vi "refs_parse_format.vi"(7 "string in":string, 8 "error in":errorcluster, 11 "str ind refs":refnum<vi>[](array[refnum])) -> (0 "error out":errorcluster)   [LabVIEW 2013]
uses:
  refs_var.vi
panel:
  out "result string":string
  out "Array":string[](array[string])
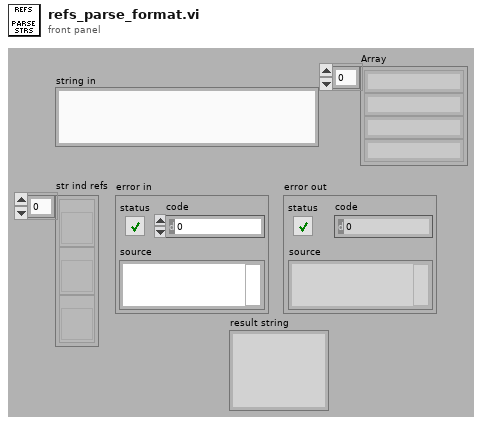
[diagram p1: front panel]
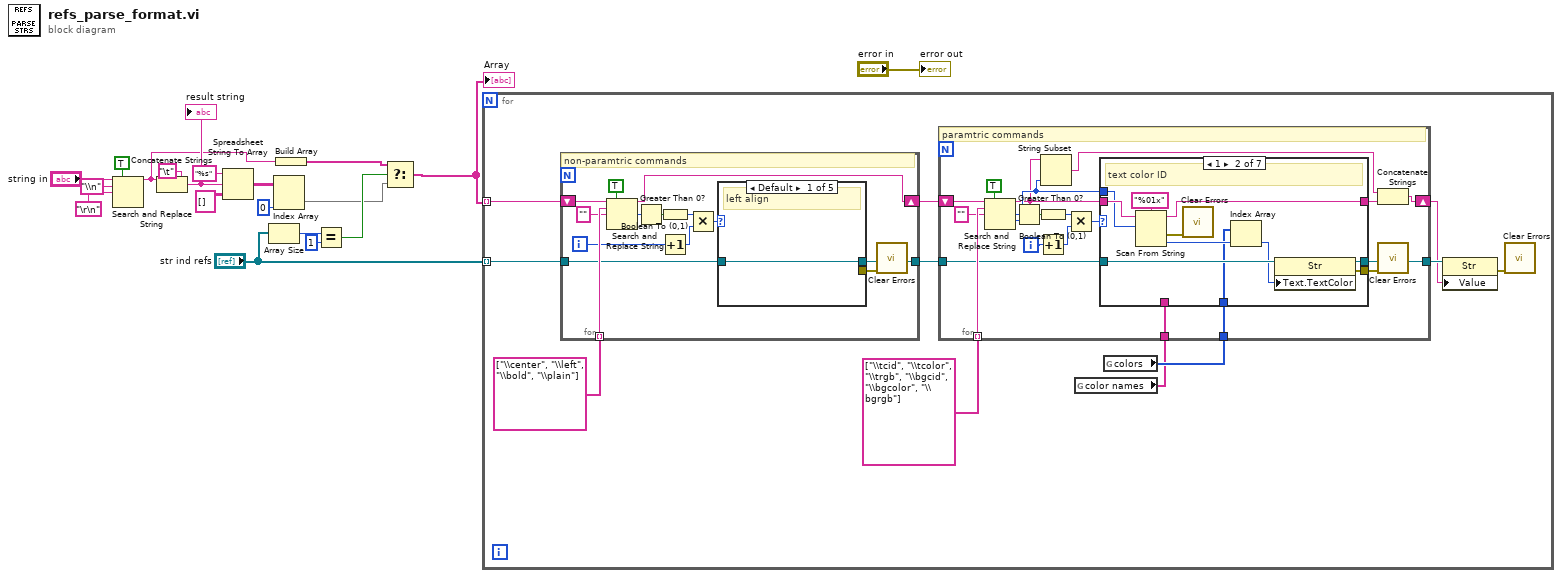
[diagram p0: block diagram]
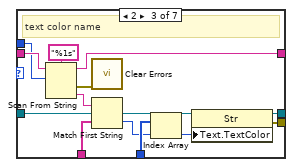
[diagram p3: hidden frame]
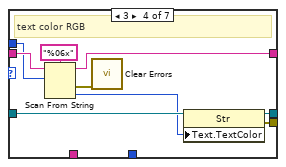
[diagram p4: hidden frame]
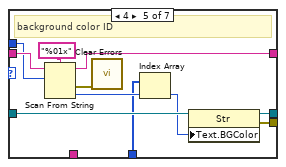
[diagram p5: hidden frame]
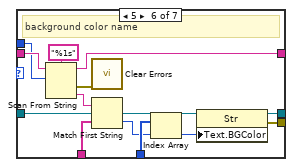
[diagram p6: hidden frame]
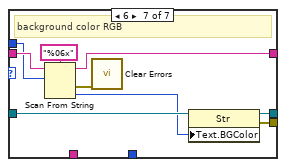
[diagram p7: hidden frame]
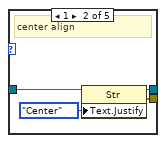
[diagram p8: hidden frame]
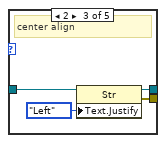
[diagram p9: hidden frame]
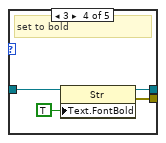
[diagram p10: hidden frame]
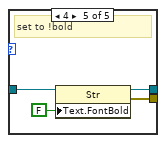
[diagram p11: hidden frame]
diagram:
  n1 = Search and Replace String(replace all?=TRUE ("replace all? (F)"), input string="string in", search string="\\n", replace string="\r\n") -> (result string=w1:string)  [unwired: 4 in, 3 out]
  n2 = Concatenate Strings(w1, "\t") -> (w4:string)
  "result string" <- w4
  n3 = Spreadsheet String To Array(format string="%s", spreadsheet string=w4, array type (2D Dbl)=string[][] []) -> (array=w13:string[][])  [unwired: 1 in]
  n4 = Array Size(array="str ind refs") -> (size(s)=w9:i32)
  n5 = Index Array(array=w13, index (col)=0 ("disabled index (col)")) -> (element=w5:string[])  [unwired: 1 in]
  n6 = Build Array(w1) -> (w3:string[])
  n7 = Equal?(x=w9, y=1) -> (x = y?=w6:bool)
  n8 = Select(t=w3, s=w6, f=w5) -> (s? t:f=w2:string[])
  "Array" <- w2
  n9 = for {
    tunnel: w2 -> [w28] mode=indexing
    tunnel: "str ind refs" -> [w30] mode=indexing
    n10 = for {
      tunnel: string[] ["\\center", "\\left", "\\bold", "\\plain"] -> [w131] mode=indexing
      tunnel: w30 -> [w122]
      tunnel: [w121] -> w27
      shift-right: [w120] -> w26
      shift-left: w28 -> [w132]
      i -> [w125]
      # "non-paramtric commands"
      n11 = Search and Replace String(replace all?=TRUE ("replace all? (F)"), input string=w132, search string=w131, replace string="" ("replace string (\"\")")) -> (result string=w120:string, number of replacements=w128:i32)  [unwired: 4 in, 2 out]
      n12 = Greater Than 0?(x=w128) -> (x > 0?=w127:bool)
      n13 = Boolean To (0,1)(Boolean=w127) -> (0, 1=w126:i16)
      n14 = Increment(x=w125) -> (x+1=w124:i32)
      n15 = Multiply(x=w126, y=w124) -> (x*y=w123:i32)
      n16 = case shown="Default" w123 {
        tunnel: w122 -> [w133 w137 w141 w145 w149]
        tunnel: [w133 w135 w139 w143 w147] -> w121
        tunnel: [_ w134 w138 w142 w146] -> w119
        frame Default {
          # "left align"
        }
        frame 1 {
          # "center align"
          n17 = property class="Str"(reference=w137, "Text.Justify"=enum16{"Left", "Center", "Right"}."Center" ("Text.Justification")) -> (reference out=w135:refnum<vi>, error out=w134:errorcluster)  [unwired: 1 in]
        }
        frame 2 {
          # "center align"
          n18 = property class="Str"(reference=w141, "Text.Justify"=enum16{"Left", "Center", "Right"}."Left" ("Text.Justification")) -> (reference out=w139:refnum<vi>, error out=w138:errorcluster)  [unwired: 1 in]
        }
        frame 3 {
          # "set to bold"
          n19 = property class="Str"(reference=w145, "Text.FontBold"=TRUE ("Text.Font:Bold")) -> (reference out=w143:refnum<vi>, error out=w142:errorcluster)  [unwired: 1 in]
        }
        frame 4 {
          # "set to !bold"
          n20 = property class="Str"(reference=w149, "Text.FontBold"=FALSE ("Text.Font:Bold")) -> (reference out=w147:refnum<vi>, error out=w146:errorcluster)  [unwired: 1 in]
        }
      }
      n21 = call <vilib>:"Clear Errors.vi"("error in (no error)"=w119) -> ()  [unwired: 6 in, 1 out]
    }
    n22 = global read "refs_var.vi" "color names"() -> (w22:string[])
    n23 = global read "refs_var.vi" "colors"() -> (w24:u32[])
    n24 = for {
      tunnel: string[] ["\\tcid", "\\tcolor", "\\trgb", "\\bgcid", "\\bgcolor", "\\bgrgb"] -> [w49] mode=indexing
      tunnel: w27 -> [w40]
      tunnel: [w39] -> w23
      shift-right: [w34] -> w21
      shift-left: w26 -> [w50]
      tunnel: w24 -> [w38]
      tunnel: w22 -> [w32]
      i -> [w43]
      # "paramtric commands"
      n25 = Search and Replace String(replace all?=TRUE ("replace all? (F)"), input string=w50, search string=w49, replace string="" ("replace string (\"\")")) -> (result string=w36:string, number of replacements=w46:i32, offset past replacement=w37:i32)  [unwired: 4 in, 1 out]
      n26 = Greater Than 0?(x=w46) -> (x > 0?=w45:bool)
      n27 = Boolean To (0,1)(Boolean=w45) -> (0, 1=w44:i16)
      n28 = Increment(x=w43) -> (x+1=w42:i32)
      n29 = String Subset(string=w36, length (rest)=w37) -> (substring=w33:string)  [unwired: 1 in]
      n30 = Multiply(x=w44, y=w42) -> (x*y=w41:i32)
      n31 = case shown="1" w41 {
        tunnel: w40 -> [w52 w63 w76 w85 w96 w109 w118]
        tunnel: [w52 w62 w75 w84 w95 w108 w117] -> w39
        tunnel: w36 -> [w51 w61 w74 w82 w93 w107 w115]
        tunnel: [w51 w54 w68 w81 w92 w101 w114] -> w35
        tunnel: w38 -> [_ w59 w73 _ w90 w106 _]
        tunnel: w37 -> [_ w56 w70 w78 w87 w103 w111]
        tunnel: w32 -> [_ _ w66 _ _ w99 _]
        tunnel: [_ w53 w64 w77 w86 w97 w110] -> w31
        frame Default {
          # "left align"
        }
        frame 1 {
          # "text color ID"
          n32 = Scan From String(format string="%01x", input string=w61, initial scan location=w56) -> (remaining string=w54:string, error out=w57:errorcluster, output 1=w60:u32)  [unwired: 2 in, 1 out]
          n33 = call <vilib>:"Clear Errors.vi"("error in (no error)"=w57) -> ()  [unwired: 6 in, 1 out]
          n34 = Index Array(array=w59, index=w60) -> (element=w58:u32)
          n35 = property class="Str"(reference=w63, "Text.TextColor"=w58) -> (reference out=w62:refnum<vi>, error out=w53:errorcluster)  [unwired: 1 in]
        }
        frame 2 {
          # "text color name"
          n36 = Scan From String(format string="%1s", input string=w74, initial scan location=w70) -> (remaining string=w68:string, error out=w71:errorcluster, output 1=w67:string)  [unwired: 2 in, 1 out]
          n37 = call <vilib>:"Clear Errors.vi"("error in (no error)"=w71) -> ()  [unwired: 6 in, 1 out]
          n38 = Match First String(2:w66, 3:w67) -> (0:w65:i32)  [unwired: 1 out]
          n39 = Index Array(array=w73, index=w65) -> (element=w72:u32)
          n40 = property class="Str"(reference=w76, "Text.TextColor"=w72) -> (reference out=w75:refnum<vi>, error out=w64:errorcluster)  [unwired: 1 in]
        }
        frame 3 {
          # "text color RGB"
          n41 = Scan From String(format string="%06x", input string=w82, initial scan location=w78) -> (remaining string=w81:string, error out=w79:errorcluster, output 1=w80:u32)  [unwired: 2 in, 1 out]
          n42 = call <vilib>:"Clear Errors.vi"("error in (no error)"=w79) -> ()  [unwired: 6 in, 1 out]
          n43 = property class="Str"(reference=w85, "Text.TextColor"=w80) -> (reference out=w84:refnum<vi>, error out=w77:errorcluster)  [unwired: 1 in]
        }
        frame 4 {
          # "background color ID"
          n44 = Scan From String(format string="%01x", input string=w93, initial scan location=w87) -> (remaining string=w92:string, error out=w88:errorcluster, output 1=w91:u32)  [unwired: 2 in, 1 out]
          n45 = call <vilib>:"Clear Errors.vi"("error in (no error)"=w88) -> ()  [unwired: 6 in, 1 out]
          n46 = Index Array(array=w90, index=w91) -> (element=w89:u32)
          n47 = property class="Str"(reference=w96, "Text.BGColor"=w89) -> (reference out=w95:refnum<vi>, error out=w86:errorcluster)  [unwired: 1 in]
        }
        frame 5 {
          # "background color name"
          n48 = Scan From String(format string="%1s", input string=w107, initial scan location=w103) -> (remaining string=w101:string, error out=w104:errorcluster, output 1=w100:string)  [unwired: 2 in, 1 out]
          n49 = call <vilib>:"Clear Errors.vi"("error in (no error)"=w104) -> ()  [unwired: 6 in, 1 out]
          n50 = Match First String(2:w99, 3:w100) -> (0:w98:i32)  [unwired: 1 out]
          n51 = Index Array(array=w106, index=w98) -> (element=w105:u32)
          n52 = property class="Str"(reference=w109, "Text.BGColor"=w105) -> (reference out=w108:refnum<vi>, error out=w97:errorcluster)  [unwired: 1 in]
        }
        frame 6 {
          # "background color RGB"
          n53 = Scan From String(format string="%06x", input string=w115, initial scan location=w111) -> (remaining string=w114:string, error out=w112:errorcluster, output 1=w113:u32)  [unwired: 2 in, 1 out]
          n54 = call <vilib>:"Clear Errors.vi"("error in (no error)"=w112) -> ()  [unwired: 6 in, 1 out]
          n55 = property class="Str"(reference=w118, "Text.BGColor"=w113) -> (reference out=w117:refnum<vi>, error out=w110:errorcluster)  [unwired: 1 in]
        }
      }
      n56 = Concatenate Strings(w33, w35) -> (w34:string)
      n57 = call <vilib>:"Clear Errors.vi"("error in (no error)"=w31) -> ()  [unwired: 6 in, 1 out]
    }
    n58 = property class="Str"(reference=w23, "Value"=w21) -> (error out=w20:errorcluster)  [unwired: 1 in, 1 out]
    n59 = call <vilib>:"Clear Errors.vi"("error in (no error)"=w20) -> ()  [unwired: 6 in, 1 out]
  }
  "error out" <- "error in"
